vi "Actor Core.vi"(8 "error in":errorcluster, 11 "LabActor in":refnum<class "OldLabActor.lvclass">) -> (0 "error out":errorcluster, 3 "Actor out":refnum<class "Actor.lvclass">)   [LabVIEW 2024, in "OldLabActor.lvclass"]
doc: "LabActor main control pannel"
uses:
  OldLabActor.lvclass
  OldLabActor.lvclass/OldLabActor.ctl
  NHMFL_Core/Libraries/Queued Listbox/Queued Listbox.xctl
  Template Module Messages/Open Item Msg/Open Item Msg.lvclass
  <vilib>/ActorFramework/Actor/Actor.lvclass
  <vilib>/ActorFramework/Stop Msg/Stop Msg.lvclass
  LabActor Messages/Start Pulse Measurements Msg/Start Measurements Command Msg.lvclass
  LabActor Messages/Stop Measurements Command Msg/Stop Measurements Command Msg.lvclass
  Controllers/Application Controller Messages/Open Waveform File Plot Msg/Open Waveform File Plot Msg.lvclass
  Plots/Plot types.ctl
  Template Module Messages/Save Configuration Msg/Save Configuration Msg.lvclass
  <vilib>/Utility/sysdir.llb/System Directory Type.ctl
  Template Module Messages/Restore Configuration Msg/Restore Configuration Msg.lvclass
  Controllers/Application Controller Messages/Pulse Acquired Result/Pulse Acquired Result.lvclass
  Controllers/Application Controller/Application Controller.lvclass
  D:/GitHub/LabActor/Controllers/Application Controller/Application Controller.lvclass
  D:/GitHub/LabActor/Controllers/Process Controller/Process Controller.lvclass
  D:/GitHub/LabActor/Worker/Worker Actor/Worker Actor.lvclass
  D:/GitHub/LabActor/Template Module/Template Module.lvclass
  C:/Program Files/National Instruments/LabVIEW 2024/vi.lib/ActorFramework/Actor/Actor.lvclass
  D:/GitHub/LabActor/Worker/Woker Interface/Worker.lvclass
  D:/GitHub/LabActor/Publish-Subscribe/Interfaces/Subscriber/Subscriber.lvclass
  D:/GitHub/LabActor/Publish-Subscribe/Interfaces/Publisher/Publisher.lvclass
  D:/GitHub/LabActor/Controllers/Interfaces/Application/Application.lvclass
  D:/GitHub/LabActor/OldLabActor Project/OldLabActor Class/OldLabActor.lvclass
panel:
  in  "About Button":bool
  in  "Clear log":bool
  out "Error log":string
  out "Monitor file":path caption="Monitor\nFile"
  in  "Exit":bool
  in  "Monitor configuration":bool
  in  "Write cfg":bool
  in  "Read cfg":bool
  in  "View XY Plot":bool
  out "Monitor Running":bool
  in  "Stop monitor":bool
  in  "Start monitor":bool
  in  "Monitor":string[](xcontrol)
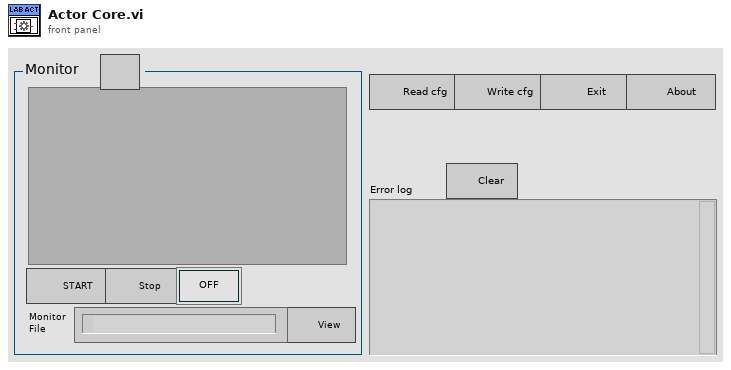
[diagram p1: front panel]
types:
  T1 = typedef "Plot types.ctl" = enum16{"Waveform Plot", "XY Plot", "Full XY"}
  T2 = typedef "System Directory Type.ctl" = i32
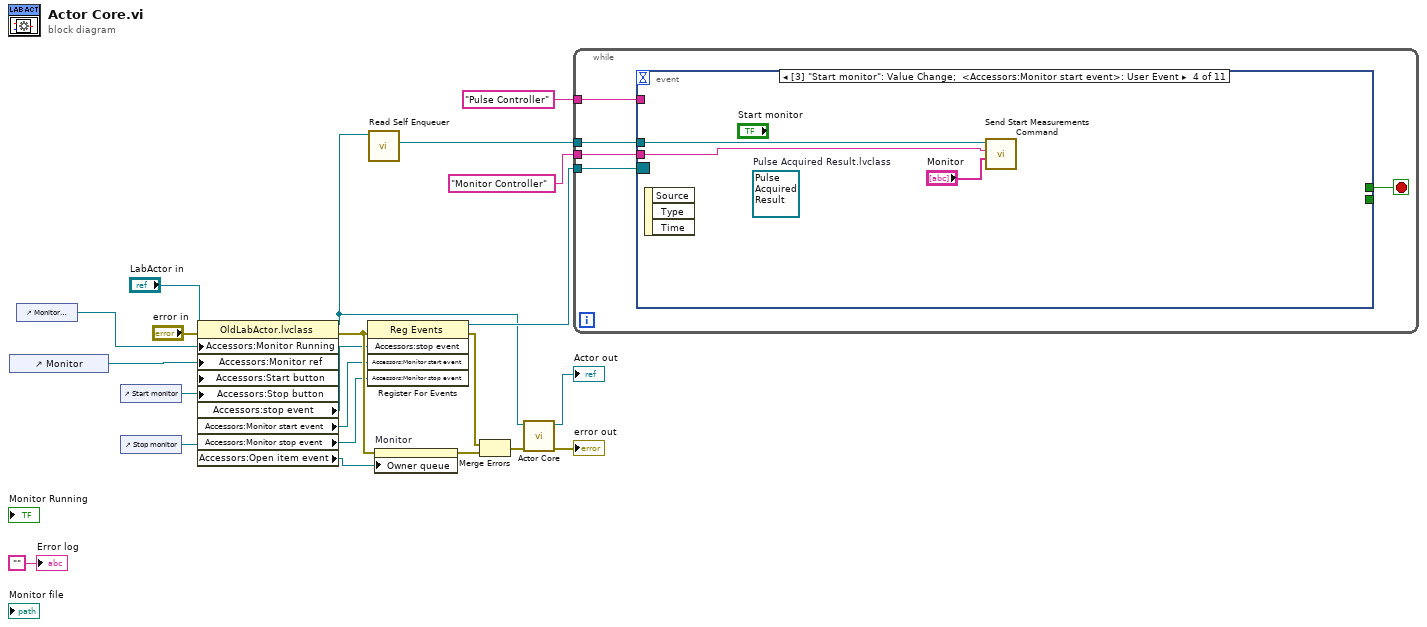
[diagram p0: block diagram]
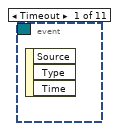
[diagram p2: hidden frame]
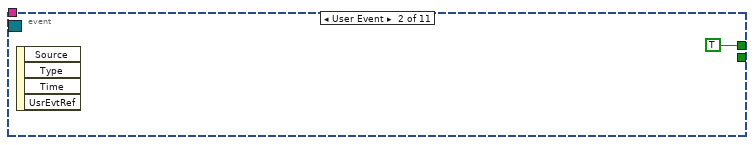
[diagram p3: hidden frame]
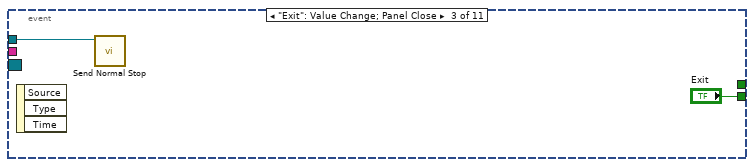
[diagram p4: hidden frame]
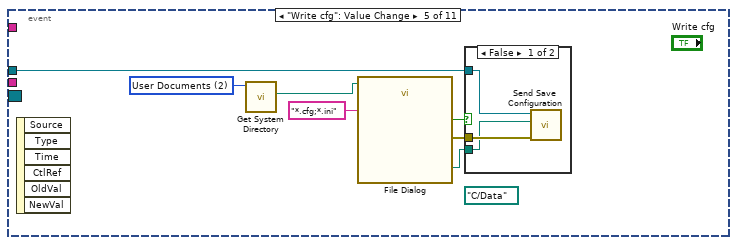
[diagram p5: hidden frame]
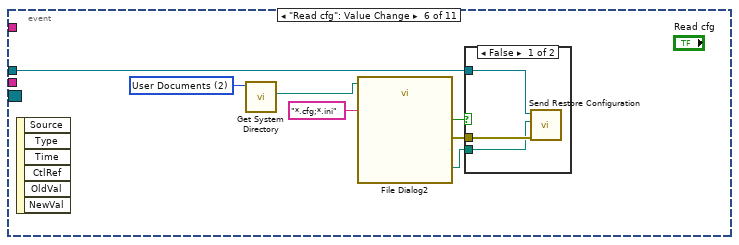
[diagram p7: hidden frame]
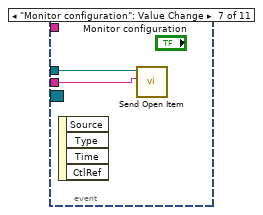
[diagram p9: hidden frame]
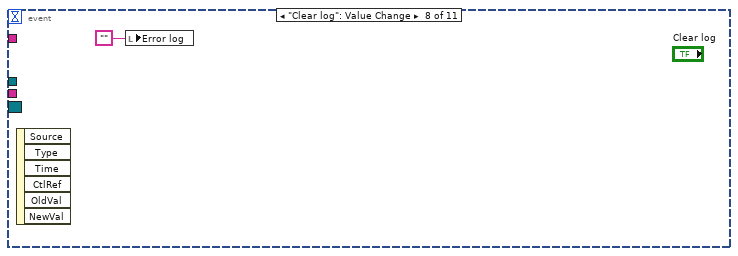
[diagram p10: hidden frame]
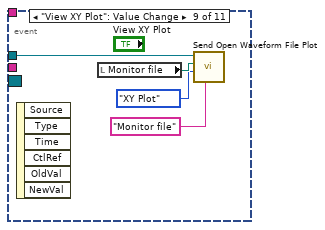
[diagram p11: hidden frame]
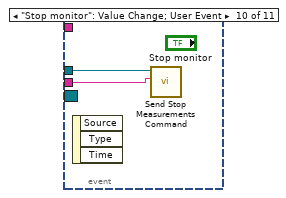
[diagram p12: hidden frame]
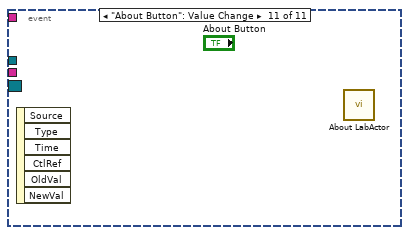
[diagram p13: hidden frame]
diagram:
  n1 = control-ref of="Monitor"() -> (w5:refnum<vi>)
  n2 = control-ref of="Monitor Running"() -> (w6:refnum<vi>)
  n3 = control-ref of="Start monitor"() -> (w3:refnum<vi>)
  n4 = control-ref of="Stop monitor"() -> (w4:refnum<vi>)
  n5 = property class="OldLabActor.lvclass"(reference="LabActor in", error in="error in", "Accessors:Monitor Running"=w6, "Accessors:Monitor ref"=w5, "Accessors:Start button"=w3, "Accessors:Stop button"=w4) -> (reference out=w12:refnum<class "OldLabActor.lvclass">, error out=w16:errorcluster, "Accessors:stop event"=w7:refnum<user-event>, "Accessors:Monitor start event"=w2:refnum<user-event>, "Accessors:Monitor stop event"=w1:refnum<user-event>, "Accessors:Open item event"=w18:refnum<user-event>)
  n6 = register-events(error in=w16, w7, w2, w1) -> (reference out=w19:refnum<event-registration>, error out=w15:errorcluster)  [unwired: 1 in]
  n7 = call <vilib>:"Read Self Enqueuer.vi"("Actor"=w12) -> ("Self Enqueuer"=w11:refnum<class "Message Enqueuer.lvclass">)  [unwired: 10 in]
  n8 = property on="Monitor" class="Queued Listbox (strict)"(error in=w16, "Owner queue"=w18) -> (error out=w17:errorcluster)  [unwired: 1 in, 1 out]
  n9 = Merge Errors(w15, w17) -> (w13:errorcluster)
  n10 = call-parent "Actor Core.vi"("error in"=w13, "Measure Object in"=w12) -> ("error out"=→"error out":errorcluster, "Actor out"=→"Actor out":refnum<class "Actor.lvclass">)  [unwired: 8 in]
  n11 = while {
    tunnel: w19 -> [w27]
    tunnel: w11 -> [w25]
    tunnel: "Monitor Controller" ("Controller name") -> [w24]
    tunnel: "Pulse Controller" ("Item name") -> [w23]
    stop <- w26 stop-if-true
    n12 = event shown="[3] \"Start monitor\": Value Change;  <Accessors:Monitor start event>: User Event" {
      selector: w27 -> [_ _ _ _ _ _ _ _ _ _ _]
      dyn-events: _ -> [_ _ _ _ _ _ _ _ _ _ _]
      timeout: _ -> [_ _ _ _ _ _ _ _ _ _ _]
      tunnel: [_ TRUE _ _ _ _ _ _ _ _ _] -> w26
      tunnel: w25 -> [_ _ w29 w32 w37 w45 w55 _ w60 w62 _]
      tunnel: [_ _ "Exit" _ _ _ _ _ _ _ _] -> _
      tunnel: w24 -> [_ _ _ w31 _ _ w54 _ _ w61 _]
      tunnel: w23 -> [_ _ _ _ _ _ _ _ _ _ _]
      event Timeout {
        n13 = event-data() -> ()  [unwired: 1 in, 3 out]
      }
      event User Event {
        n14 = event-data() -> ()  [unwired: 1 in, 4 out]
      }
      event "Exit": Value Change; Panel Close {
        n15 = event-data() -> ()  [unwired: 1 in, 3 out]
        n16 = call <vilib>:"Send Normal Stop.vi"("Message Enqueuer"=w29) -> ()  [unwired: 10 in, 1 out]
      }
      event "Start monitor": Value Change; User Event {
        (unwired) refnum<class "Pulse Acquired Result.lvclass"> refnum  # Pulse Acquired Result.lvclass
        n17 = event-data() -> ()  [unwired: 1 in, 3 out]
        n18 = call "Send Start Measurements Command.vi"("Objects"="Monitor", "Controller name"=w31, "Message Enqueuer"=w32) -> ()  [unwired: 7 in, 2 out]
      }
      event "Write cfg": Value Change {
        w35 = T2 2 items=["User Home"=0, "User Desktop"=1, "User Documents"=2, "User Application Data"=3, "User Preferences"=4, "User Temporary"=5, "Public Documents"=6, "Public Application Data"=7, "Public Preferences"=8, "Public Cache"=13, "System Core Libraries"=9, "System Installed Libraries"=10, "Application Files"=11, "Boot Volume Root"=12] ("system directory type")
        (unwired) path "C:/Data" ("start path")
        n19 = event-data() -> ()  [unwired: 1 in, 6 out]
        n20 = call <vilib>:"Get System Directory.vi"("system directory type"=w35) -> ("system directory"=w34:path)  [unwired: 10 in]
        n21 = call "File Dialog"("start path"=w34, "pattern (all files)"="*.cfg;*.ini") -> ("selected path"=w39:path, "cancelled"=w40:bool, "error out"=w36:errorcluster)  [unwired: 10 in, 1 out]
        n22 = case shown="False" w40 {
          tunnel: w39 -> [w41 _]
          tunnel: w37 -> [w43 _]
          tunnel: w36 -> [w42 _]
          frame False {
            n23 = call "Send Save Configuration.vi"("error in (no error)"=w42, "File path"=w41, "Message Enqueuer"=w43) -> ()  [unwired: 7 in, 2 out]
          }
          frame True {
          }
        }
      }
      event "Read cfg": Value Change {
        w47 = T2 2 items=["User Home"=0, "User Desktop"=1, "User Documents"=2, "User Application Data"=3, "User Preferences"=4, "User Temporary"=5, "Public Documents"=6, "Public Application Data"=7, "Public Preferences"=8, "Public Cache"=13, "System Core Libraries"=9, "System Installed Libraries"=10, "Application Files"=11, "Boot Volume Root"=12] ("system directory type")
        n24 = event-data() -> ()  [unwired: 1 in, 6 out]
        n25 = call <vilib>:"Get System Directory.vi"("system directory type"=w47) -> ("system directory"=w46:path)  [unwired: 10 in]
        n26 = call "File Dialog2"("start path"=w46, "pattern (all files)"="*.cfg;*.ini") -> ("selected path"=w50:path, "cancelled"=w44:bool, "error out"=w48:errorcluster)  [unwired: 10 in, 1 out]
        n27 = case shown="False" w44 {
          tunnel: w50 -> [w51 _]
          tunnel: w45 -> [w53 _]
          tunnel: w48 -> [w52 _]
          frame False {
            n28 = call "Send Restore Configuration.vi"("error in (no error)"=w52, "File path"=w51, "Message Enqueuer"=w53) -> ()  [unwired: 7 in, 2 out]
          }
          frame True {
          }
        }
      }
      event "Monitor configuration": Value Change {
        n29 = event-data() -> ()  [unwired: 1 in, 4 out]
        n30 = call "Send Open Item.vi"("Item name"=w54, "Message Enqueuer"=w55) -> ()  [unwired: 8 in, 2 out]
      }
      event "Clear log": Value Change {
        n31 = event-data() -> ()  [unwired: 1 in, 6 out]
        n32 = local write "Error log"("" ("Error log")) -> ()
      }
      event "View XY Plot": Value Change {
        n33 = event-data() -> ()  [unwired: 1 in, 6 out]
        n34 = local read "Monitor file"() -> (w59:path)
        n35 = call "Send Open Waveform File Plot.vi"("Plot group"="Monitor file" ("Control Name"), "Plot type"=Plot_types."XY Plot", "File Path Control"=w59, "Message Enqueuer"=w60) -> ()  [unwired: 6 in, 2 out]
      }
      event "Stop monitor": Value Change; User Event {
        n36 = event-data() -> ()  [unwired: 1 in, 3 out]
        n37 = call "Send Stop Measurements Command.vi"("Measurement Controller"=w61, "Message Enqueuer"=w62) -> ()  [unwired: 8 in, 2 out]
      }
      event "About Button": Value Change {
        n38 = event-data() -> ()  [unwired: 1 in, 6 out]
        n39 = call "About LabActor.vi"() -> ()  [unwired: 11 in, 1 out]
      }
    }
  }
  "Error log" <- "" ("Error log")
